vi "Hardware In - NI 9758-1 (PFI-LS).vi"(11 "FPGA Ref":T1) -> ()   [LabVIEW 2015, in "ECS-RT.lvlib"]
uses:
  ECS-RT.lvlib
  Typedefs/FPGA Refs/Generic FPGA Ref.ctl
  <vilib>/Utility/error.llb/Error Cluster From Error Code.vi
  <vilib>/rvi/errors/niLvFpgaAdjustHostInterfaceError.vi
  <vilib>/rvi/interface/nirviReadWriteControl/nirviReadWriteControl.xnode
  <vilib>/rvi/interface/Simulation/niFpgaSimulationCallBeginRW.vi
  NiFpgaLv.dll
  ECS-Shared.lvlib
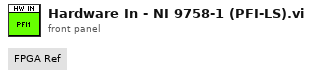
[diagram p1: front panel]
types:
  T1 = typedef "ECS-Shared.lvlib/Generic FPGA Ref.ctl" = refnum<k20>
  T2 = cluster{"ModulePresent":bool, "Fault1":u8, "Fault2":u8, "HardwareRev":u8, "FirmwareRev":u8}
  T3 = cluster{"LS1Open":bool, "LS2Open":bool, "LS3Open":bool, "LS4Open":bool, "PFI1Open":bool, "PFI2Open":bool, "PFI3Open":bool, "PFI4Open":bool}
  T4 = cluster{"LS1Short":bool, "LS2Short":bool, "LS3Short":bool, "LS4Short":bool, "PFI1Short":bool, "PFI2Short":bool, "PFI3Short":bool, "PFI4Short":bool}
  T5 = cluster{"ModulePresent":bool, "Hardware Rev":string, "Firmware Rev":u8}
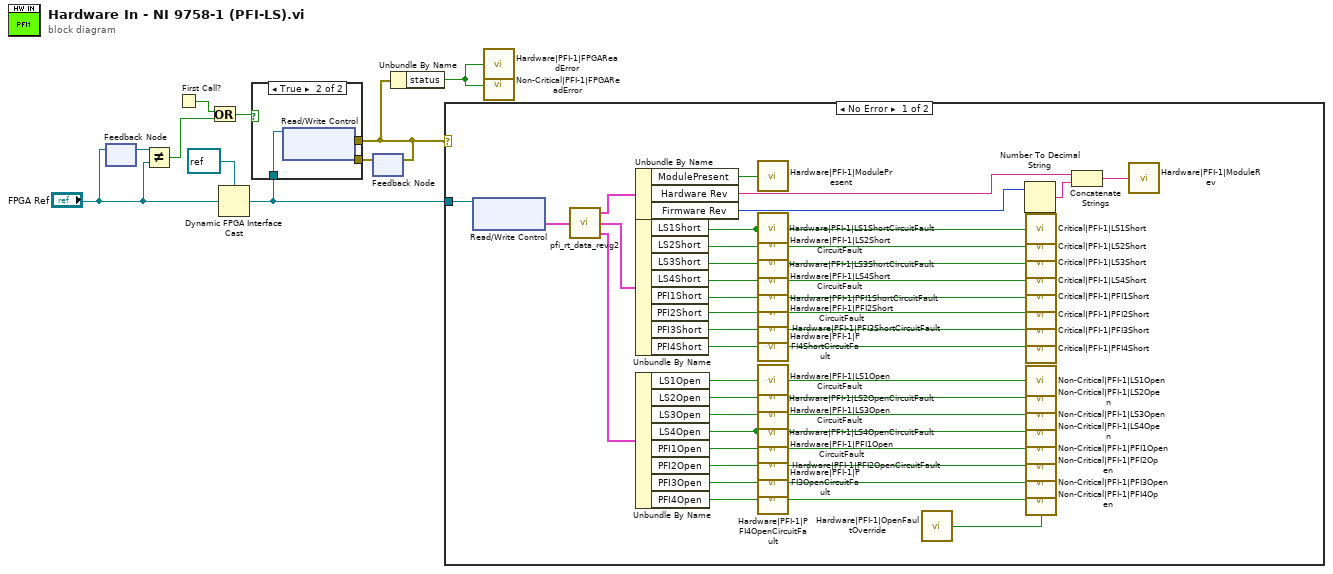
[diagram p0: block diagram]
diagram:
  n1 = feedback #1() -> (w9:T1)  [unwired: 1 in]
  n2 = feedback-in #1("FPGA Ref") -> ()
  n3 = Not Equal?(x=w9, y="FPGA Ref") -> (x != y?=w10:bool)
  n4 = First Call?() -> (First Call?: T/F=w8:bool)
  n5 = Or(x=w8, y=w10) -> (x .or. y?=w7:bool)
  n6 = Dynamic FPGA Interface Cast(Session In=refnum<k20> refnum ("FPGA VI Reference Out"), Type="FPGA Ref") -> (Session Out=w3:refnum<k20>)
  n7 = feedback #2() -> (w6:errorcluster)  [unwired: 1 in]
  n8 = case shown="True" w7 {
    tunnel: [w11 w13] -> w2
    tunnel: w6 -> [w11 _]
    tunnel: w3 -> [_ w12]
    frame False {
    }
    frame True {
      n9 = xnode "Read/Write Control"("FPGA VI Reference In"=w12) -> ("error out"=w13:errorcluster)  [unwired: 1 in, 2 out]
    }
  }
  n10 = feedback-in #2(w2) -> ()
  n11 = Unbundle By Name(w2) -> ("status"=w1:bool)
  n12 = case shown="No Error" w2 {
    tunnel: w3 -> [w14 _]
    frame No Error {
      n13 = xnode "Read/Write Control"("FPGA VI Reference In"=w14) -> ("PFI-1.Data"=w15:T2)  [unwired: 1 in, 2 out]
      n14 = call <vilib>:"pfi_rt_data_revg2.vi"("PFIDataFromFPGA"=w15) -> ("Non Critical Faults"=w17:T3, "Critical Faults"=w16:T4, "PFIData"=w19:T5)  [unwired: 2 in]
      n15 = Unbundle By Name(w19) -> ("ModulePresent"=w38:bool, "Hardware Rev"=w39:string, "Firmware Rev"=w40:u8)
      n16 = Unbundle By Name(w16) -> ("LS1Short"=w23:bool, "LS2Short"=w22:bool, "LS3Short"=w21:bool, "LS4Short"=w20:bool, "PFI1Short"=w24:bool, "PFI2Short"=w25:bool, "PFI3Short"=w26:bool, "PFI4Short"=w27:bool)
      n17 = Unbundle By Name(w17) -> ("LS1Open"=w28:bool, "LS2Open"=w29:bool, "LS3Open"=w30:bool, "LS4Open"=w31:bool, "PFI1Open"=w32:bool, "PFI2Open"=w33:bool, "PFI3Open"=w34:bool, "PFI4Open"=w35:bool)
      n18 = call "Hardware|PFI-1|ModulePresent"("Value"=w38) -> ()
      n19 = call "Hardware|PFI-1|LS1ShortCircuitFault"("Value"=w23) -> ()
      n20 = call "Hardware|PFI-1|LS2ShortCircuitFault"("Value"=w22) -> ()
      n21 = call "Hardware|PFI-1|LS3ShortCircuitFault"("Value"=w21) -> ()
      n22 = call "Hardware|PFI-1|LS4ShortCircuitFault"("Value"=w20) -> ()
      n23 = call "Hardware|PFI-1|PFI1ShortCircuitFault"("Value"=w24) -> ()
      n24 = call "Hardware|PFI-1|PFI2ShortCircuitFault"("Value"=w25) -> ()
      n25 = call "Hardware|PFI-1|PFI3ShortCircuitFault"("Value"=w26) -> ()
      n26 = call "Hardware|PFI-1|PFI4ShortCircuitFault"("Value"=w27) -> ()
      n27 = call "Hardware|PFI-1|LS1OpenCircuitFault"("Value"=w28) -> ()
      n28 = call "Hardware|PFI-1|LS2OpenCircuitFault"("Value"=w29) -> ()
      n29 = call "Hardware|PFI-1|LS3OpenCircuitFault"("Value"=w30) -> ()
      n30 = call "Hardware|PFI-1|LS4OpenCircuitFault"("Value"=w31) -> ()
      n31 = call "Hardware|PFI-1|PFI1OpenCircuitFault"("Value"=w32) -> ()
      n32 = call "Hardware|PFI-1|PFI2OpenCircuitFault"("Value"=w33) -> ()
      n33 = call "Hardware|PFI-1|PFI3OpenCircuitFault"("Value"=w34) -> ()
      n34 = call "Hardware|PFI-1|PFI4OpenCircuitFault"("Value"=w35) -> ()
      n35 = call "Hardware|PFI-1|OpenFaultOverride"() -> ("Value"=w18:bool)
      n36 = Number To Decimal String(number=w40) -> (decimal integer string=w37:string)  [unwired: 1 in]
      n37 = call "Critical|PFI-1|LS1Short"("Fault"=w23) -> ()  [unwired: 2 in]
      n38 = call "Critical|PFI-1|LS2Short"("Fault"=w22) -> ()  [unwired: 2 in]
      n39 = call "Critical|PFI-1|LS3Short"("Fault"=w21) -> ()  [unwired: 2 in]
      n40 = call "Critical|PFI-1|LS4Short"("Fault"=w20) -> ()  [unwired: 2 in]
      n41 = call "Critical|PFI-1|PFI1Short"("Fault"=w24) -> ()  [unwired: 2 in]
      n42 = call "Critical|PFI-1|PFI2Short"("Fault"=w25) -> ()  [unwired: 2 in]
      n43 = call "Critical|PFI-1|PFI3Short"("Fault"=w26) -> ()  [unwired: 2 in]
      n44 = call "Critical|PFI-1|PFI4Short"("Fault"=w27) -> ()  [unwired: 2 in]
      n45 = call "Non-Critical|PFI-1|LS1Open"("Fault"=w28, "Override (F)"=w18) -> ()  [unwired: 1 in]
      n46 = call "Non-Critical|PFI-1|LS2Open"("Fault"=w29, "Override (F)"=w18) -> ()  [unwired: 1 in]
      n47 = call "Non-Critical|PFI-1|LS3Open"("Fault"=w30, "Override (F)"=w18) -> ()  [unwired: 1 in]
      n48 = call "Non-Critical|PFI-1|LS4Open"("Fault"=w31, "Override (F)"=w18) -> ()  [unwired: 1 in]
      n49 = call "Non-Critical|PFI-1|PFI1Open"("Fault"=w32, "Override (F)"=w18) -> ()  [unwired: 1 in]
      n50 = call "Non-Critical|PFI-1|PFI2Open"("Fault"=w33, "Override (F)"=w18) -> ()  [unwired: 1 in]
      n51 = call "Non-Critical|PFI-1|PFI3Open"("Fault"=w34, "Override (F)"=w18) -> ()  [unwired: 1 in]
      n52 = call "Non-Critical|PFI-1|PFI4Open"("Fault"=w35, "Override (F)"=w18) -> ()  [unwired: 1 in]
      n53 = Concatenate Strings(w39, w37) -> (w36:string)
      n54 = call "Hardware|PFI-1|ModuleRev"("Value"=w36) -> ()
    }
    frame Error {
    }
  }
  n55 = call "Hardware|PFI-1|FPGAReadError"("Value"=w1) -> ()
  n56 = call "Non-Critical|PFI-1|FPGAReadError"("Fault"=w1) -> ()  [unwired: 2 in]
